vi "Continuous Triggered Acquisition.vi"() -> ()   [LabVIEW 2021]
doc: "Use this VI as a template to design an application that acquires multiple records of data from the NI PXIe-5170R/5171R."
uses:
  <instrlib>/_niInstr/Multirecord Acquisition/Interface/v1/Host/Public/Requested Record Info.ctl
  <instrlib>/_niInstr/Multirecord Acquisition/Interface/v1/Host/Public/Full Record Status.ctl
  <instrlib>/_niInstr/Multirecord Acquisition/Interface/v1/Host/Public/Record State.ctl
  <instrlib>/_niInstr/Multirecord Acquisition/Interface/v1/Host/Public/Record Status.ctl
  <vilib>/FPGAPlugInAG/PXIe-5172 (8CH - 410T)/niLvFpga_Open_PXIe-5172 (8CH - 410T).vi
  <vilib>/rvi/interface/common/dynamic/niFpgaDynamicAddResources.vi
  <vilib>/FPGAPlugInAG/Dynamic/niLvFpga_Close_Dynamic.vi
  <vilib>/rvi/interface/nirviOpenFPGA/nirviOpenFPGA.xnode
  FPGA Bitfiles/5172 Multirecord Acquisition custom trigger.lvbitx
  <vilib>/rvi/interface/nirviCloseFPGA/nirviCloseFPGA.xnode
  Device Session/Device Session.lvclass
  <instrlib>/_niInstr/Multirecord Acquisition/Interface/v1/Host/niInstr Multirecord Acquisition v1 Host.lvclass
panel:
  out "record status 2":T1
  out "records done 2":u64
  out "current record status 2":T3
  out "requested records info 2":T4[](array[typedef])
  out "Waveform 1":T5(graph)
  out "overflow occurred 2":bool
  in  "Trigger Settings":T6={"channel"=0, "Center"=0.0, "Range"=0.2999999523162842}
  out "overflow occurred":bool
  in  "Stop":bool
  out "current record status":T3
  out "records done":u64
  out "record status":T1
  in  "pretrigger samples":u64=100
  out "Waveform 0":T5(graph)
  in  "number of samples":u64=5000
  in  "channels to configure":string="0"
  out "error out":errorcluster
  out "requested records info":T4[](array[typedef])
  in  "RIO Device":tag="PXI1Slot8"
  # "RIO Device"
  # "Channels"
  # "Acquisition Settings"
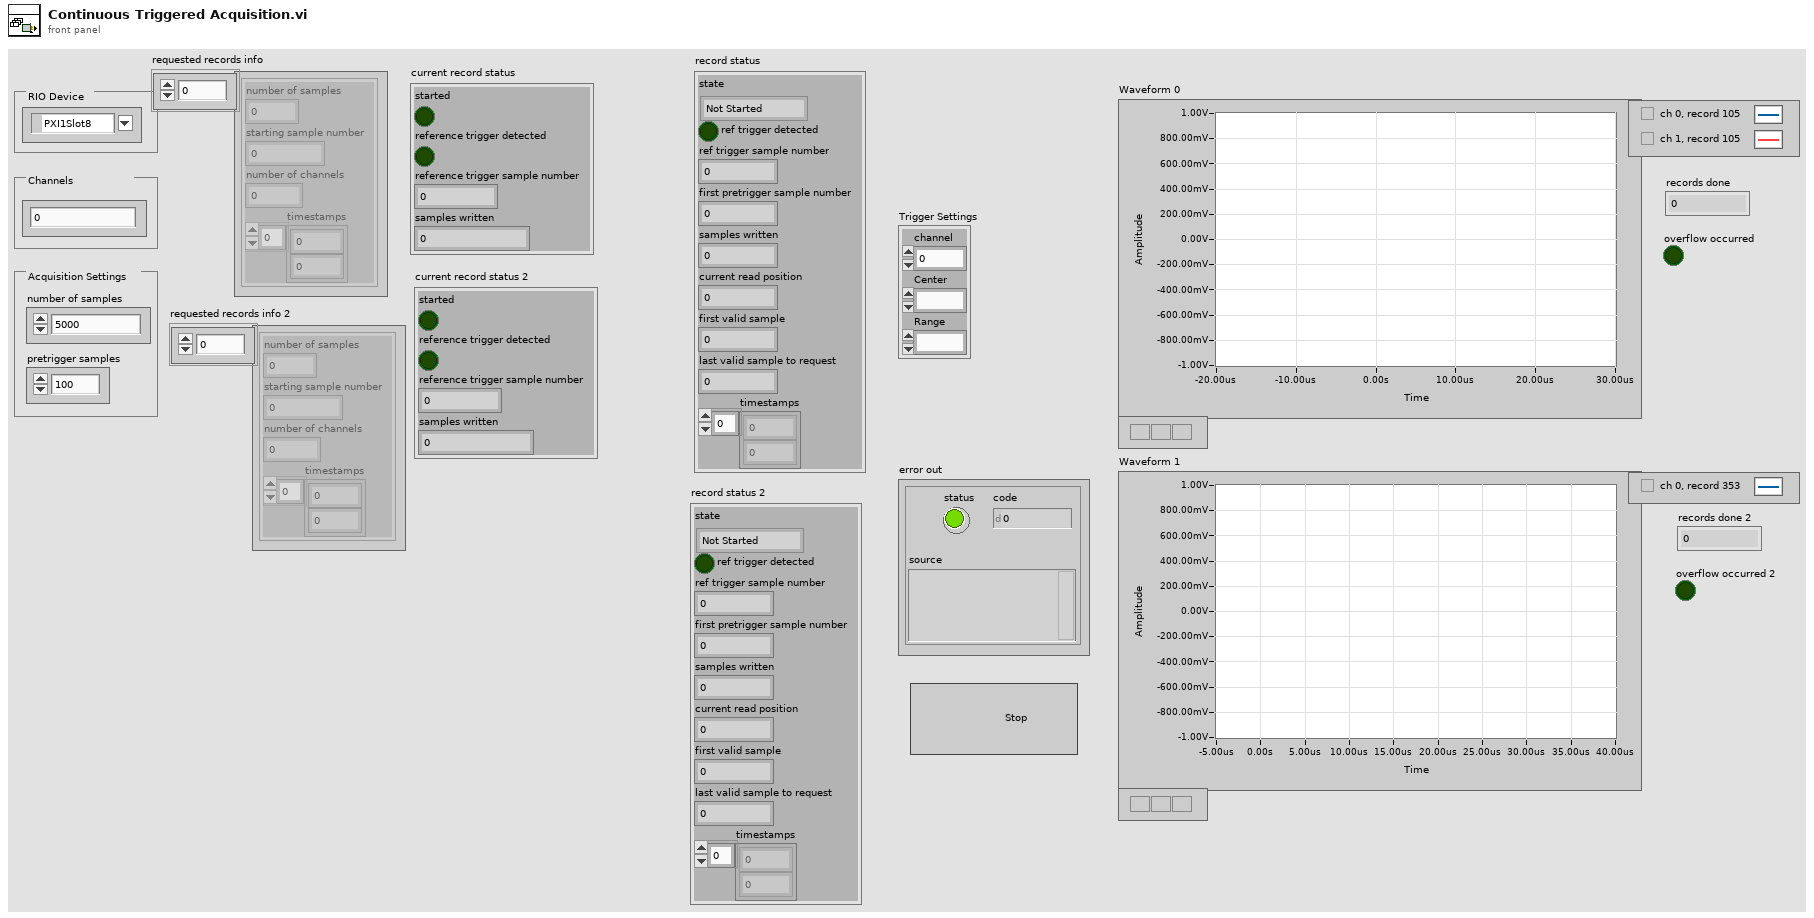
[diagram p1: front panel]
types:
  T1 = typedef "niInstr Multirecord Acquisition v1 Host.lvclass/Full Record Status.ctl" = cluster{"state":T2, "ref trigger detected":bool, "ref trigger sample number":u64, "first pretrigger sample number":u64, "samples written":u64, "current read position":u64, "first valid sample":u64, "last valid sample to request":u64, "timestamps":u64[]}
  T2 = typedef "niInstr Multirecord Acquisition v1 Host.lvclass/Record State.ctl" = enum16{"Not Started", "Being Acquired", "Completed", "Overwritten"}
  T3 = typedef "niInstr Multirecord Acquisition v1 Host.lvclass/Record Status.ctl" = cluster{"started":bool, "reference trigger detected":bool, "reference trigger sample number":u64, "samples written":u64}
  T4 = typedef "niInstr Multirecord Acquisition v1 Host.lvclass/Requested Record Info.ctl" = cluster{"number of samples":u64, "starting sample number":u64, "number of channels":u64, "timestamps":u64[]}
  T5 = cluster{"relativeX":dbl, "sample rate":dbl, "data in":dbl[]}[]
  T6 = cluster{"channel":u8, "Center":fxp<+/-,24,1>, "Range":fxp<+,24,1>}
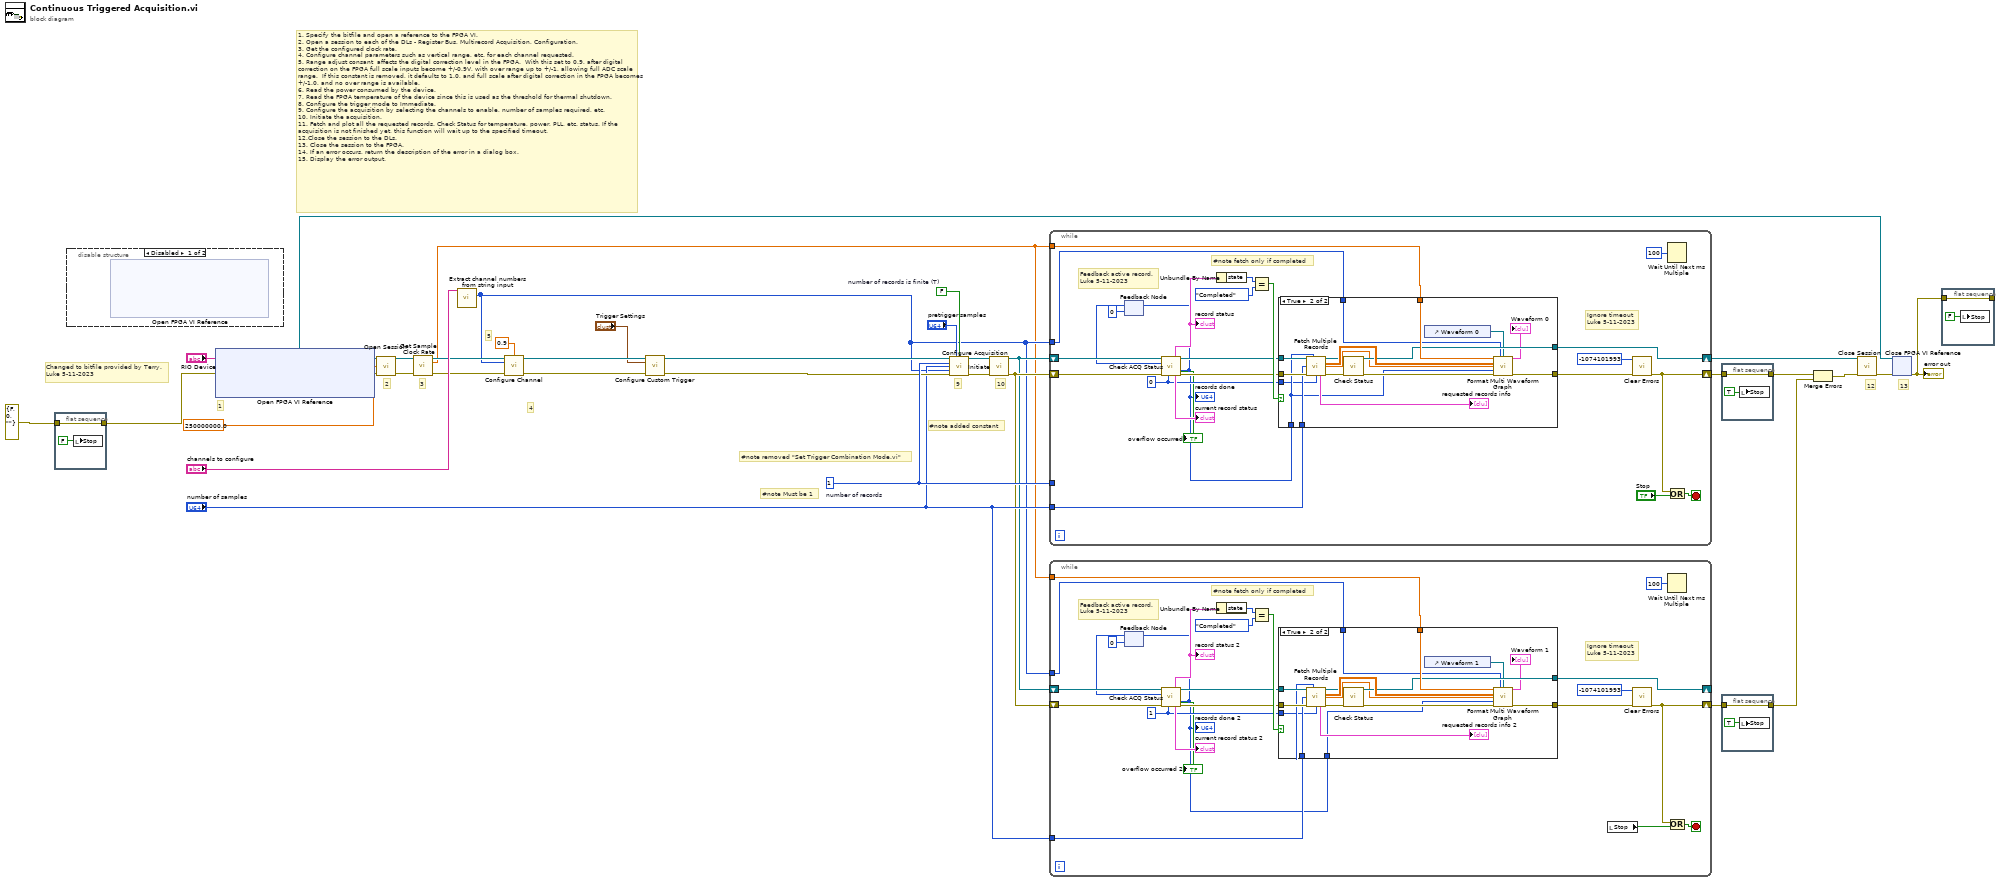
[diagram p0: block diagram]
diagram:
  w22 = 250000000.0 items=["250 MHz"=250000000.0, "200 MHz"=200000000.0, "150 MHz"=150000000.0] ("onboard sample clock rate")
  w24 = u64 1  # number of records
  w20 = FALSE  # number of records is finite (T)
  # "Changed to bitfile provided by Terry.\nLuke 5-11-2023"
  # "#note removed \"Set Trigger Combination Mode.vi\""
  # "#note Must be 1"
  # "#note added constant"
  # "5"
  # "13"
  # "12"
  # "10"
  # "9"
  # "4"
  # "3"
  # "1"
  # "2"
  # "1. Specify the bitfile and open a reference to the FPGA VI.\n2. Open a session to each of the DLs - Register Bus, Multirecord Acquisition, Configuration.\n3. Get the configured clock rate.\n4. Configure channel parameters such as vertical range, etc. for each channel requested.\n5. Range adjust consant  affects the digital correction level in the FPGA.  With this set to 0.9, after digital correction on the FPGA full scale inputs become +/-0.9V, with over range up to +/-1, allowing full ADC scale range.  If this constant is removed, it defaults to 1.0, and full scale after digital correction in the FPGA becomes +/-1.0, and no over range is available.\n6. Read the power consumed by the device.\n7. Read the FPGA temperature of the device since this is used as the threshold for thermal shutdown.\n8. Configure the trigger mode to Immediate.\n9. Configure the acquisition by selecting the channels to enable, number of samples required, etc.\n10. Initiate the acquisition.\n11. Fetch and plot all the requested records. Check Status for temperature, power, PLL, etc. status. If the acquisition is not finished yet, this function will wait up to the specified timeout.\n12.Close the session to the DLs.\n13. Close the session to the FPGA.\n14. If an error occurs, return the description of the error in a dialog box.\n15. Display the error output."
  n1 = flat-sequence {
    tunnel: [w36] -> w2
    tunnel: errorcluster {"status"=FALSE, "code"=0, "source"=""} ("error in") -> [w36]
    frame #0 {
      n2 = local write "Stop"(FALSE ("Stop")) -> ()
    }
  }
  n3 = disable-structure shown="Disabled" {
    frame Disabled {
      n4 = xnode "Open FPGA VI Reference"() -> ()  [unwired: 2 in, 2 out]
    }
    frame Enabled {
    }
  }
  n5 = xnode "Open FPGA VI Reference"("error in"=w2, "resource name"="RIO Device") -> ("FPGA VI Reference Out"=w26:refnum<k20>, "error out"=w14:errorcluster)
  n6 = call "Open Session.vi"("FPGA VI Reference In"=w26, "adc clock rate (Hz)"=w22, "error in"=w14) -> ("device session out"=w30:refnum<class "Device Session.lvclass">, "error out"=w31:errorcluster)  [unwired: 11 in]
  n7 = call "Get Sample Clock Rate.vi"("device session in"=w30, "error in"=w31) -> ("device session out"=w29:refnum<class "Device Session.lvclass">, "sample clock rate (Hz)"=w9:dbl, "error out"=w28:errorcluster)  [unwired: 11 in]
  n8 = call "Extract channel numbers from string input.vi"("channel input"="channels to configure") -> ("array of chans"=w10:u32[])  [unwired: 13 in, 1 out]
  n9 = call "Configure Channel.vi"("device session in"=w29, "range adjust"=0.9, "channels"=w10, "error in"=w28) -> ("device session out"=w19:refnum<class "Device Session.lvclass">, "error out"=w18:errorcluster)  [unwired: 10 in]
  n10 = call "Configure Custom Trigger.vi"("device session in"=w19, "Trigger Settings"="Trigger Settings", "error in"=w18) -> ("device session out"=w17:refnum<class "Device Session.lvclass">, "error out"=w16:errorcluster)  [unwired: 11 in]
  n11 = call "Configure Acquisition.vi"("device session in"=w17, "pretrigger samples"="pretrigger samples", "number of records is finite (T)"=w20, "number of records"=w24, "number of samples"="number of samples", "channels to store"=w10, "error in"=w16) -> ("device session out"=w35:refnum<class "Device Session.lvclass">, "error out"=w34:errorcluster)  [unwired: 6 in, 1 out]
  n12 = call "Initiate.vi"("device session in"=w35, "error in"=w34) -> ("device session out"=w11:refnum<class "Device Session.lvclass">, "error out"=w12:errorcluster)  [unwired: 12 in]
  n13 = while {
    tunnel: "number of samples" -> [w44]
    tunnel: w9 -> [w43]
    shift-right: [w41] -> w7
    shift-left: w12 -> [w47]
    shift-right: [w61] -> w32
    shift-left: w11 -> [w48]
    tunnel: w10 -> [w45]
    tunnel: w24 -> [_]
    stop <- w60 stop-if-true
    w49 = u8 0 ("channel")
    # "Ignore timeout\nLuke 5-11-2023"
    # "Feedback active record.\nLuke 5-11-2023"
    # "#note fetch only if completed"
    n14 = feedback #1(u64 0 ("record number")) -> (w39:u64)
    n15 = call "Check ACQ Status.vi"("device session in"=w48, "record number"=w39, "error in"=w47, "channel"=w49) -> ("record status"=w57:T1, "device session out"=w51:refnum<class "Device Session.lvclass">, "records done"=w38:u64, "overflow occurred"=→"overflow occurred":bool, "current record status"=→"current record status":T3, "error out"=w50:errorcluster)  [unwired: 6 in]
    "record status" <- w57
    "records done" <- w38
    n16 = feedback-in #1(w38) -> ()
    n17 = Unbundle By Name(w57) -> ("state"=w56:T2)
    n18 = Equal?(x=w56, y=Record_State."Completed" ("state")) -> (x = y?=w54:bool)
    n19 = case shown="True" w54 {
      tunnel: w43 -> [_ w79]
      tunnel: [w62 w77] -> w61
      tunnel: w45 -> [_ w76]
      tunnel: [w63 w71] -> w59
      tunnel: w51 -> [w62 w70]
      tunnel: w50 -> [w63 w69]
      tunnel: w44 -> [_ w68]
      tunnel: w38 -> [_ w67]
      tunnel: w49 -> [_ w64]
      frame False {
      }
      frame True {
        n20 = call "Fetch Multiple Records.vi"("device session in"=w70, "starting record"=w67, "number of samples"=w68, "error in"=w69, "channel"=w64) -> ("device session out"=w72:refnum<class "Device Session.lvclass">, "data"=w80:dbl[][], "relativeX (samples)"=w75:dbl[], "requested records info"=→"requested records info":T4[], "error out"=w74:errorcluster)  [unwired: 6 in]
        n21 = call "Check Status.vi"("device session in"=w72, "error in"=w74) -> ("device session out"=w77:refnum<class "Device Session.lvclass">, "error out"=w73:errorcluster)  [unwired: 12 in]
        n22 = control-ref of="Waveform 0"() -> (w66:refnum<vi>)
        n23 = call "Format Multi Waveform Graph.vi"("sample rate (Hz)"=w79, "array of chans"=w76, "waveform graph"=w66, "data in"=w80, "relativeX (samples)"=w75, "start record number"=w67, "error in"=w73) -> ("waveform out"=→"Waveform 0":T5, "error out"=w71:errorcluster)  [unwired: 7 in]
      }
    }
    n24 = call <vilib>:"Clear Errors.vi"("error in (no error)"=w59, "specific error code to clear (0: all)"=-1074101993) -> ("error out"=w41:errorcluster)  [unwired: 4 in, 1 out]
    n25 = Wait Until Next ms Multiple(millisecond multiple=u32 100) -> ()  [unwired: 1 out]
    n26 = Compound Arithmetic op=OR(w41, "Stop") -> (w60:bool)
  }
  n27 = while {
    tunnel: "number of samples" -> [w88]
    tunnel: w9 -> [w87]
    shift-right: [w85] -> w6
    shift-left: w12 -> [w91]
    shift-right: [w104] -> _
    shift-left: w11 -> [w92]
    tunnel: w10 -> [w89]
    stop <- w103 stop-if-true
    w93 = u8 1 ("channel")
    # "Ignore timeout\nLuke 5-11-2023"
    # "Feedback active record.\nLuke 5-11-2023"
    # "#note fetch only if completed"
    n28 = feedback #2(u64 0 ("record number")) -> (w82:u64)
    n29 = call "Check ACQ Status.vi"("device session in"=w92, "record number"=w82, "error in"=w91, "channel"=w93) -> ("record status"=w100:T1, "device session out"=w95:refnum<class "Device Session.lvclass">, "records done"=w81:u64, "overflow occurred"=→"overflow occurred 2":bool, "current record status"=→"current record status 2":T3, "error out"=w94:errorcluster)  [unwired: 6 in]
    "record status 2" <- w100
    "records done 2" <- w81
    n30 = feedback-in #2(w81) -> ()
    n31 = Unbundle By Name(w100) -> ("state"=w99:T2)
    n32 = Equal?(x=w99, y=Record_State."Completed" ("state")) -> (x = y?=w97:bool)
    n33 = case shown="True" w97 {
      tunnel: w87 -> [_ w122]
      tunnel: [w105 w120] -> w104
      tunnel: w89 -> [_ w119]
      tunnel: [w106 w114] -> w102
      tunnel: w95 -> [w105 w113]
      tunnel: w94 -> [w106 w112]
      tunnel: w88 -> [_ w111]
      tunnel: w81 -> [_ w110]
      tunnel: w93 -> [_ w107]
      frame False {
      }
      frame True {
        n34 = call "Fetch Multiple Records.vi"("device session in"=w113, "starting record"=w110, "number of samples"=w111, "error in"=w112, "channel"=w107) -> ("device session out"=w115:refnum<class "Device Session.lvclass">, "data"=w123:dbl[][], "relativeX (samples)"=w118:dbl[], "requested records info"=→"requested records info 2":T4[], "error out"=w117:errorcluster)  [unwired: 6 in]
        n35 = call "Check Status.vi"("device session in"=w115, "error in"=w117) -> ("device session out"=w120:refnum<class "Device Session.lvclass">, "error out"=w116:errorcluster)  [unwired: 12 in]
        n36 = control-ref of="Waveform 1"() -> (w109:refnum<vi>)
        n37 = call "Format Multi Waveform Graph.vi"("sample rate (Hz)"=w122, "array of chans"=w119, "waveform graph"=w109, "data in"=w123, "relativeX (samples)"=w118, "start record number"=w110, "error in"=w116) -> ("waveform out"=→"Waveform 1":T5, "error out"=w114:errorcluster)  [unwired: 7 in]
      }
    }
    n38 = local read "Stop"() -> (w83:bool)
    n39 = call <vilib>:"Clear Errors.vi"("error in (no error)"=w102, "specific error code to clear (0: all)"=-1074101993) -> ("error out"=w85:errorcluster)  [unwired: 4 in, 1 out]
    n40 = Wait Until Next ms Multiple(millisecond multiple=u32 100) -> ()  [unwired: 1 out]
    n41 = Compound Arithmetic op=OR(w85, w83) -> (w103:bool)
  }
  n42 = flat-sequence {
    tunnel: [w124] -> w8
    tunnel: w7 -> [w124]
    frame #0 {
      n43 = local write "Stop"(TRUE ("Stop")) -> ()
    }
  }
  n44 = flat-sequence {
    tunnel: [w126] -> w4
    tunnel: w6 -> [w126]
    frame #0 {
      n45 = local write "Stop"(TRUE ("Stop")) -> ()
    }
  }
  n46 = Merge Errors(w8, w4) -> (w5:errorcluster)
  n47 = call "Close Session.vi"("device session in"=w32, "error in"=w5) -> ("error out"=w25:errorcluster)  [unwired: 13 in]
  n48 = xnode "Close FPGA VI Reference"("FPGA VI Reference In"=w26, "error in"=w25) -> ("error out"=w3:errorcluster)
  "error out" <- w3
  n49 = flat-sequence {
    tunnel: [w128] -> _
    tunnel: w3 -> [w128]
    frame #0 {
      n50 = local write "Stop"(FALSE ("Stop")) -> ()
    }
  }
